vi "MGCC_EnergyMgmt_main.vi"   [LabVIEW 2016]
uses:
  Finite State Machine (He Yin)/Sub-VIs/MGCC_FntStaMach_gobal.vi
  Sub-VIs/SwitchCombo.vi
  Sub-VIs/LoadCombo.vi
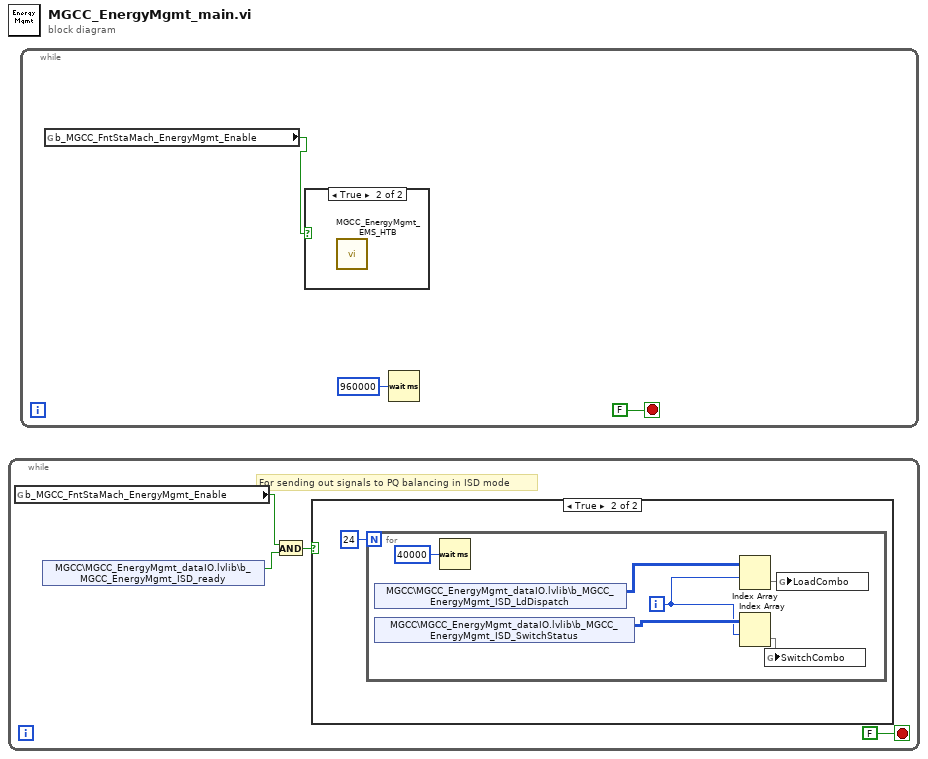
[diagram p0: block diagram]
diagram:
  n1 = while {
    stop <- FALSE stop-if-true
    # "For sending out signals to PQ balancing in ISD mode"
    n2 = global read "MGCC_FntStaMach_gobal.vi" "b_MGCC_FntStaMach_EnergyMgmt_Enable"() -> (w1:bool)
    n3 = shared-variable "MGCC\\MGCC_EnergyMgmt_dataIO.lvlib\\b_MGCC_EnergyMgmt_ISD_ready"() -> (w4:bool)  [unwired: 1 in, 1 out]
    n4 = And(x=w1, y=w4) -> (x .and. y?=w3:bool)
    n5 = case shown="True" w3 {
      frame False {
      }
      frame True {
        n6 = for {
          N: 24 -> [_]
          i -> [w8]
          n7 = shared-variable "MGCC\\MGCC_EnergyMgmt_dataIO.lvlib\\b_MGCC_EnergyMgmt_ISD_LdDispatch"() -> (w10:i32[][])  [unwired: 1 in, 1 out]
          n8 = shared-variable "MGCC\\MGCC_EnergyMgmt_dataIO.lvlib\\b_MGCC_EnergyMgmt_ISD_SwitchStatus"() -> (w9:i32[][])  [unwired: 1 in, 1 out]
          n9 = Wait (ms)(milliseconds to wait=u32 40000) -> ()  [unwired: 1 out]
          n10 = Index Array(array=w10, index (row)=w8) -> (element=w7:i32[])  [unwired: 1 in]
          n11 = Index Array(array=w9, index (row)=w8) -> (element=w6:i32[])  [unwired: 1 in]
          n12 = global write "SwitchCombo.vi" "SwitchCombo"(w6) -> ()
          n13 = global write "LoadCombo.vi" "LoadCombo"(w7) -> ()
        }
      }
    }
  }
  n14 = while {
    stop <- FALSE stop-if-true
    n15 = global read "MGCC_FntStaMach_gobal.vi" "b_MGCC_FntStaMach_EnergyMgmt_Enable"() -> (w12:bool)
    n16 = case shown="True" w12 {
      frame False {
      }
      frame True {
        n17 = call "MGCC_EnergyMgmt_EMS_HTB.vi"() -> ()  [unwired: 12 in]
      }
    }
    n18 = Wait (ms)(milliseconds to wait=u32 960000) -> ()  [unwired: 1 out]
  }
